vi "Get Refnum Information.vi"(8 "error in (no error)":errorcluster, 11 "variant":variant) -> (0 "error out":errorcluster, 1 "VI Server generic type":T1, 2 "strict type":variant, 3 "reference type":T2)   [LabVIEW 2024, in "NI_Data Type.lvlib"]
doc: "<p>Retrieves <a href=\"nihelplauncher://docs/csh?context=lvcore_lvconcepts_refnum_controls_and_indicators\">refnum</a> information from the data type stored in <strong>variant</strong>. This VI returns an error if <strong>variant</strong> does not contain a refnum.</p>"
uses:
  NI_Data Type.lvlib
  Refnum Type.ctl
  VI Server Generic Type.ctl
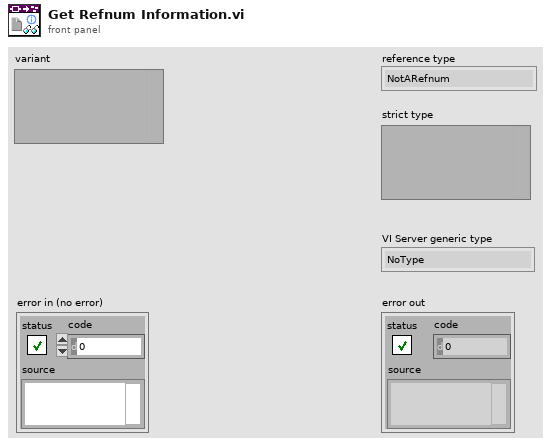
[diagram p1: front panel]
types:
  T1 = typedef "NI_Data Type.lvlib/VI Server Generic Type.ctl" = enum16{"NoType", "\tkLVObjApp=0x1", "\tkLVObjVI", "\tkLVObjGeneric", "\tkLVObjDecoration", "\tkLVObjText", "\tkLVObjControl", "\tkLVObjColorBox", "\tkLVObjBoolean", "\tkLVObjRefNum", "\tkLVObjVariant", "\tkLVObjPath", "\tkLVObjListBox", "\tkLVObjTable", "\tkLVObjArray", "\tkLVObjPicture", "\tkLVObjOleContainer", "\tkLVObjNumeric", "\tkLVObjDigital", "\tkLVObjNamedNumeric", "\tkLVObjColorRamp", "\tkLVObjSlide", "\tkLVObjGraphOrChart", "\tkLVObjWaveformChart", "\tkLVObjWaveformGraph", "\tkLVObjIntensityChart", "\tkLVObjIntensityGraph", "\tkLVObjString", "\tkLVObjIOName", "\tkLVObjComboBox", "\tkLVObjCluster", "\tkLVObjPanel", "\tkLVObjKnob", "\tkLVObjNumWithScale", "\tkLVObjRing", "\tkLVObjEnum", "\tkLVObjGObject", "\tkLVObjPlot", "\tkLVObjCursor", "\tkLVObjNumericText", "\tkLVObjScale", "\tkLVObjColorScale", "\tkLVObjGraphScale", "\tkLVObjColorGraphScale", "\tkLVObjTypedRefNum", "\tkLVObjOldKnobScale", "\tkLVObjMCListbox", "\tkLVObjMeasureData", "\tkLVObjDSCTag", "\tkLVObjDAQName", "\tkLVObjVISAName", "\tkLVObjIVIName", "\tkLVObjSlideScale", "\tkLVObjTabControl", "\tkLVObjPage", "\tkLVObjTabArrayTabControl", "\tkLVObjConPane", "\tkLVObjDAQMXName", "\tkLVObjVIRefNum", "\tkLVObjLVObjRefNum", "\tkLVObjAbsTime", "\tkLVObjDigitalTable", "\tkLVObjUnused", "\tkLVObjUnused2", "\tkLVObjSCLControl", "\tkLVObjSubPanel", "\tkLVObjTreeControl", "\tkLVObjGenClassTagRef", "\tkLVObjGenClassRef", "\tkLVObjRotaryColorScale", "\tkLVObjPlugInDDOControl", "\tkLVObjPlugInDDOClassHolder", "\tkLVObjRadClusControl", "\tkLVObjProject", "\tkLVObjProjectItem", "\tkLVObjPane", "\tkLVObjSplitterBar", "\tkLVObjProjectBuildItem", "\tkLVObjPixmap", "\tkLVObjFacadeVI", "\tkLVObjLibrary", "\tkLVObjVariable", "\tkLVObjPropertyBag", "\tkLVObjXYGraph", "\tkLVObjScene", "\tkLVObjUDClassLibrary", "\tkLVObjUDClassClone", "\tkLVObjMethodVI", "\tkLVObjXCtlLibrary", "\tkLVObjXNodeLibrary", "\tkLVObjScroll", "\tkLVObjLVTarget", "\tkLVObjMixedGraph", "\tkLVObjProvider", "\tkLVObjCopyOperation", "\tkLVObjTargetItem", "\tkLVObjProjectItemType", "\tkLVObjCopyItem", "\tkLVObjCopyConflict", "\tkLVObjCopyExpert", "\tkLVObjSceneGraphDisp", "\tkLVObjPolyVI", "\tkLVObjLVClassDDO", "kLVObjDiagram=0x4000", "\tkLVObjTerminal", "\tkLVObjConstant", "\tkLVObjPathConstant", "\tkLVObjArrayConstant", "\tkLVObjNumericConstant", "\tkLVObjDigitalNumConstant", "\tkLVObjNamedNumericConstant", "\tkLVObjStringConstant", "\tkLVObjClusterConstant", "\tkLVObjFixedConstant", "\tkLVObjControlTerminal", "\tkLVObjFormulaParameter", "\tkLVObjGlobal", "\tkLVObjLocal", "\tkLVObjRightShiftRegister", "\tkLVObjFunction", "\tkLVObjSubVI", "\tkLVObjCallByRef", "\tkLVObjUnitCast", "\tkLVObjStructure", "\tkLVObjLoop", "\tkLVObjMultiframeStructure", "\tkLVObjSequence", "\tkLVObjCaseSelector", "\tkLVObjFormula", "\tkLVObjGrowableFunction", "\tkLVObjBuildClusterArray", "\tkLVObjCompoundArithmetic", "\tkLVObjIndexArray", "\tkLVObjBuildArray", "\tkLVObjNamedBundler", "\tkLVObjCIN", "\tkLVObjCallLibrary", "\tkLVObjObjectFunction", "\tkLVObjProperty", "\tkLVObjInvoke", "\tkLVObjNode", "\tkLVObjBooleanConstant", "\tkLVObjBlockDiagram", "\tkLVObjRingConstant", "\tkLVObjEnumConstant", "\tkLVObjTunnel", "\tkLVObjLoopTunnel", "\tkLVObjSequenceLocal", "\tkLVObjComparison", "\tkLVObjReadWriteFile", "\tkLVObjTypeCast", "\tkLVObjFlattenUnflattenString", "\tkLVObjGPIBReadWrite", "\tkLVObjForLoop", "\tkLVObjWhileLoop", "\tkLVObjScriptNode", "\tkLVObjArrayToCluster", "\tkLVObjFormatScanString", "\tkLVObjWire", "\tkLVObjProbe", "\tkLVObjInnerTerminal", "\tkLVObjLeftShiftRegister", "\tkLVObjPolySubVI", "\tkLVObjPropItem", "\tkLVObjIONameConstant", "\tkLVObjDSCTagConstant", "\tkLVObjDAQNameConstant", "\tkLVObjVISANameConstant", "\tkLVObjIVINameConstant", "\tkLVObjColorBoxConstant", "\tkLVObjControlRefConstant", "\tkLVObjClassSpecifierConstant", "\tkLVObjConfNode", "\tkLVObjMasterWizard", "\tkLVObjStateDiagWizard", "\tkLVObjOuterTerminal", "\tkLVObjDAQMXNameConstant", "\tkLVObjEventStructure", "\tkLVObjFlatSequence", "\tkLVObjGenClassTagRefConstant", "\tkLVObjAbsTimeConstant", "\tkLVObjExternalNode", "\tkLVObjSubWizard", "\tkLVObjScriptNodeParameter", "\tkLVObjStatVIRef", "\tkLVObjComboBoxConstant", "\tkLVObjTimedLoop", "\tkLVObjGenClassDeepCopy", "\tkLVObjGenClassTagFlat", "\tkLVObjGenClassTagFlatRefConstant", "\tkLVObjGenClassFlat", "\tkLVObjSimDiagram", "\tkLVObjCompDiagram", "\tkLVObjSimNode", "\tkLVObjSimDCO", "\tkLVObjBundler", "\tkLVObjUnbundler", "\tkLVObjNamedUnbundler", "\tkLVObjFlatSeqFrame", "\tkLVObjFlatSeqInTun", "\tkLVObjFlatSeqOutTun", "\tkLVObjRefNumConst", "\tkLVObjFlattenString", "\tkLVObjPolySelector", "\tkLVObjXNode", "\tkLVObjSelectorTunnel", "\tkLVObjCommentNode", "\tkLVObjSdfDiagram", "\tkLVObjSDFCompDiagram", "\tkLVObjSdfNode", "\tkLVObjSdfDCO", "\tkLVObjFileDialog", "\tkLVObjTLDCO", "\tkLVObjTimeSeqFrame", "\tkLVObjTimeFlatSequence", "\tkLVObjTimedSequence", "\tkLVObjXDataNode", "\tkLVObjCodeWizard", "\tkLVObjMathScriptNode", "\tkLVObjMathScriptNodeParameter", "\tkLVObjLVClassBDConst"}
  T2 = typedef "NI_Data Type.lvlib/Refnum Type.ctl" = enum16{"NotARefnum", "UnknownRefnum", "Generic", "Datalog", "ByteStream", "Device", "Occurence", "TCPNetConnection", "Auto", "Menu", "Imaq", "Hardware", "DataSocket", "Visa", "IVI", "UDPNetConnection", "Notifier", "Queue", "Irda", "EventReg", "DotNet", "UserEvent", "Callback", "UNUSED_EMPTY_POSITION", "BlueToothNetConnection", "LVObjApp", "LVObjVI", "LVObjUnknown", "GenericClass", "UserDefinedRefnumTag", "DataValue", "RT FIFO", "TDMS File", "PythonSessionRefnum"}
  T3 = enum16{"Generic", "Datalog", "ByteStream", "Device", "Occurence", "TCPNetConnection", "OldVisa", "Auto", "LVObj", "Menu", "OldIVI", "Imaq", "Hardware", "DataSocket", "Visa", "IVI", "UDPNetConnection", "Notifier", "Queue", "Irda", "GenClass", "GenClassTag", "DAQmx", "EventReg", "DotNet", "UserEvent", "GenClassDeepCopy", "Callback", "GenClassFlatten", "GenClassTagFlatten", "LVClassInst", "BlueToothNetConnection", "DataValue", "RT FIFO", "TDMS File", "PythonSessionRefnum"}
  T4 = enum16{"Generic", "Datalog", "ByteStream", "Device", "Occurence", "TCPNetConnection", "OldVisa", "Auto", "LVObj", "Menu", "OldIVI", "Imaq", "Hardware", "DataSocket", "Visa", "IVI", "UDPNetConnection", "Notifier", "Queue", "Irda", "GenClass", "GenClassTag", "DAQmx", "EventReg", "DotNet", "UserEvent", "GenClassDeepCopy", "Callback", "GenClassFlatten", "GenClassTagFlatten", "LVClassInst", "BlueToothNetConnection", "DataValue", "RT FIFO", "TDMS File"}
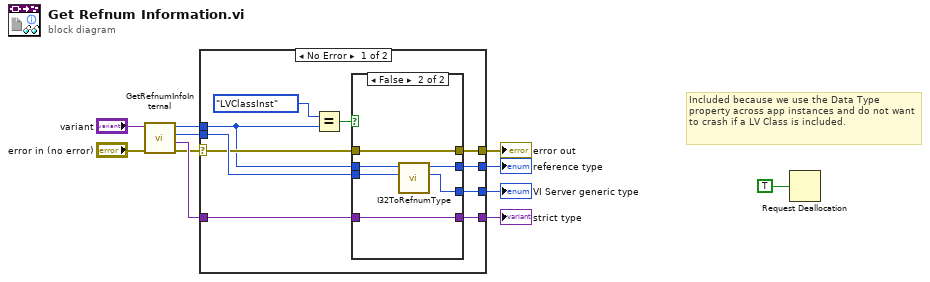
[diagram p0: block diagram]
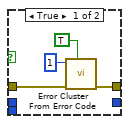
[diagram p2: hidden frame]
diagram:
  # "Included because we use the Data Type property across app instances and do not want to crash if a LV Class is included."
  n1 = call "GetRefnumInfoInternal.vi"("error in (no error)"="error in (no error)", "Variant"="variant") -> ("error out"=w2:errorcluster, "StrictType"=w6:variant, "subKind"=w7:i32, "Refnum Kind"=w5:T3)  [unwired: 5 in, 1 out]
  n2 = case shown="No Error" w2 {
    selector: w2 -> [w15 w32]
    tunnel: [w21 _] -> w11
    tunnel: [w20 _] -> w10
    tunnel: [w19 _] -> w8
    tunnel: w7 -> [w18 _]
    tunnel: w6 -> [w17 _]
    tunnel: w5 -> [w14 _]
    tunnel: [w16 w32] -> w3
    frame No Error {
      n3 = Equal?(x=T4."LVClassInst" ("Refnum Kind"), y=w14) -> (x = y?=w12:bool)
      n4 = case shown="False" w12 {
        tunnel: w14 -> [_ w30]
        tunnel: [_ w28] -> w21
        tunnel: w18 -> [_ w29]
        tunnel: [_ w31] -> w20
        tunnel: w17 -> [_ w31]
        tunnel: [_ w27] -> w19
        tunnel: w15 -> [w25 w26]
        tunnel: [w23 w26] -> w16
        frame True {
          n5 = call "Error Cluster From Error Code.vi"("show call chain? (False)"=TRUE, "error in (no error)"=w25, "error code (0)"=1) -> ("error out"=w23:errorcluster)  [unwired: 6 in]
        }
        frame False {
          n6 = call "I32ToRefnumType.vi"("Subkind"=w29, "Kind"=w30) -> ("VI Server Generic Type"=w27:T1, "ReferenceType"=w28:T2)  [unwired: 8 in]
        }
      }
    }
    frame Error {
    }
  }
  "error out" <- w3
  "strict type" <- w10
  "reference type" <- w11
  "VI Server generic type" <- w8
  n7 = Request Deallocation(TRUE ("flag")) -> ()
